vi "Unit Tester.vi"() -> ()   [LabVIEW 2012]
doc: "This VI lists all VI's in the various \"unit tests\" directories located under the directory in which this VI resides. It is then possible to run the unit tests or open the test panels. Unit tests must have a compatible connector pane for a call by reference. This user interface will be replaced by a more scripting oriented alternative in due time."
uses:
  t_Unit Tester States.ctl
panel:
  in  "open selected":bool
  in  "unit test call type":refnum<vi>
  in  "reinitialize":bool
  in  "abort":bool
  in  "run all":bool
  in  "unit tests":i32[](listbox)
  in  "stop":bool
  in  "run selected":bool
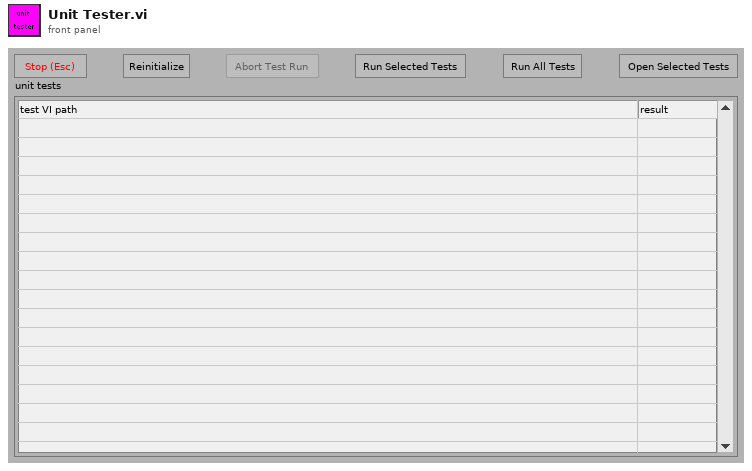
[diagram p1: front panel]
types:
  T1 = typedef "t_Unit Tester States.ctl" = enum16{"empty queue", "adjust size", "run", "open", "initialize", "cleanup", "stop"}
  T2 = enum32{"Bad", "Idle", "Run top level", "Running"}
  T3 = typedef "eventvkey.ctl" = enum16{"ASCII", "Enter", "Return", "Shift", "Ctrl", "Alt", "Cmd", "Opt", "Caps", "NumLock", "Clear", "Break", "Up", "Down", "Left", "Right", "Insert", "Delete", "Home", "End", "PageUp", "PageDown", "Escape", "Help", "Pause", "ScrollLock", "F1", "F2", "F3", "F4", "F5", "F6", "F7", "F8", "F9", "F10", "F11", "F12", "F13", "F14", "F15", "F16", "F17", "F18", "F19", "F20", "F21", "F22", "F23", "F24", "Play", "VolumeUp", "VolumeDown", "Mute", "Two Byte Char"}
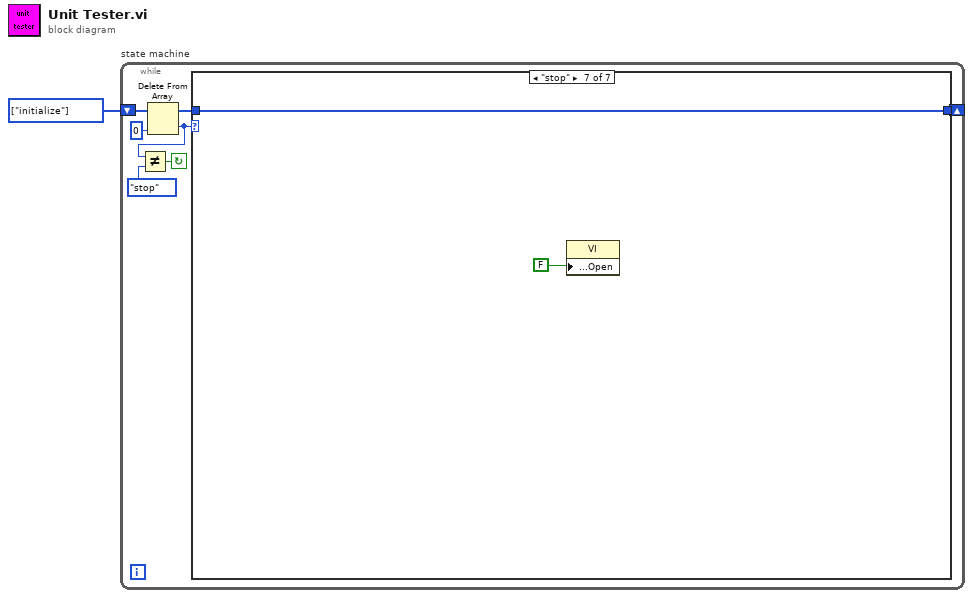
[diagram p0: block diagram]
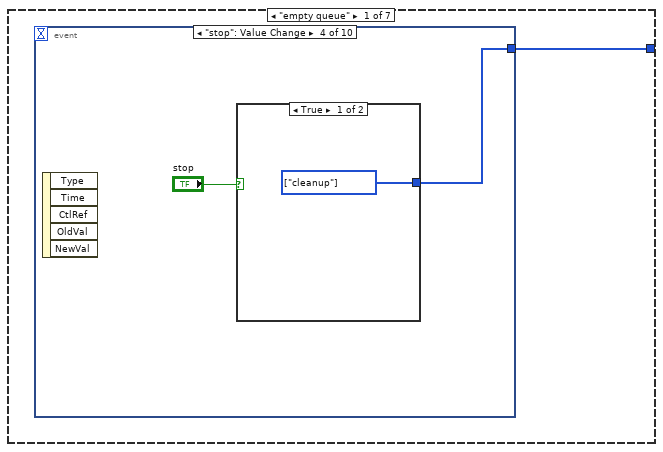
[diagram p2: hidden frame]
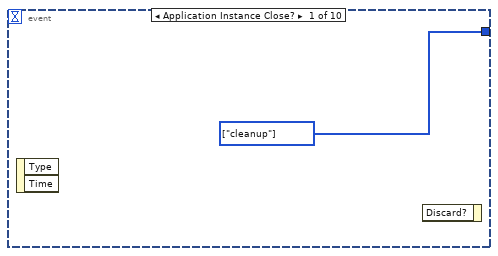
[diagram p3: hidden frame]
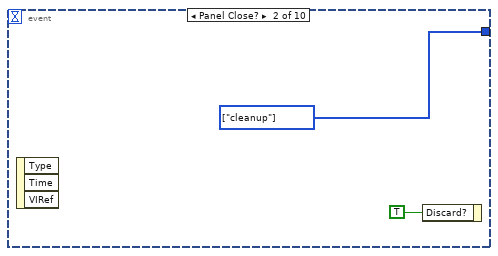
[diagram p4: hidden frame]
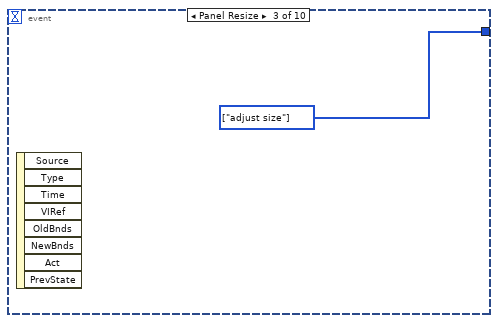
[diagram p5: hidden frame]
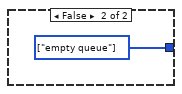
[diagram p6: hidden frame]
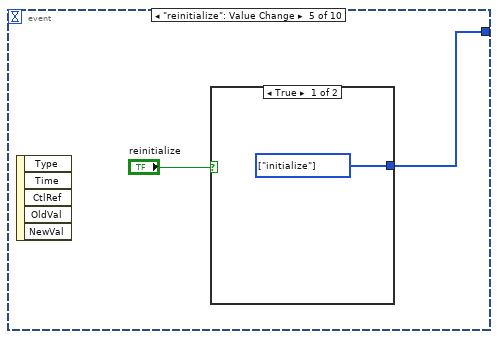
[diagram p7: hidden frame]
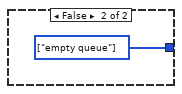
[diagram p8: hidden frame]
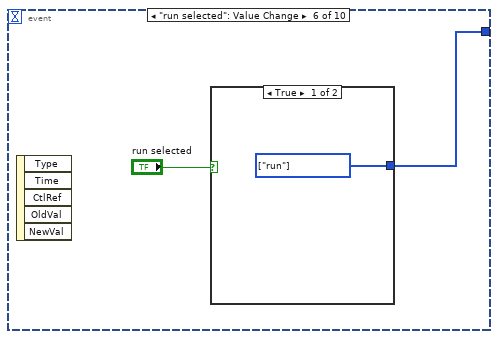
[diagram p9: hidden frame]
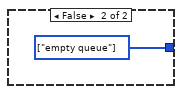
[diagram p10: hidden frame]
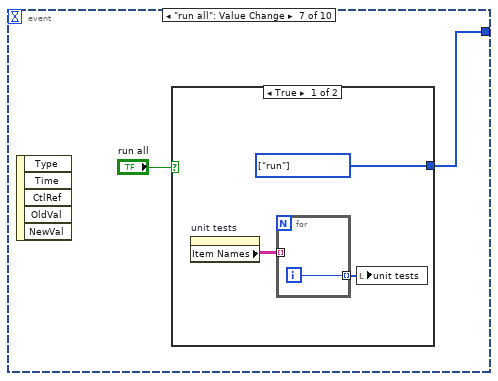
[diagram p11: hidden frame]
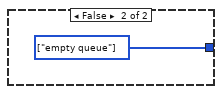
[diagram p12: hidden frame]
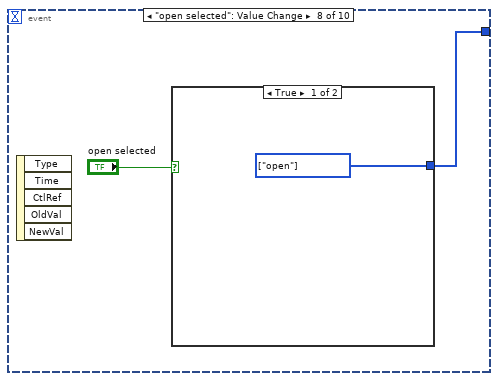
[diagram p13: hidden frame]
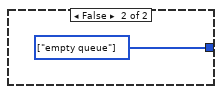
[diagram p14: hidden frame]
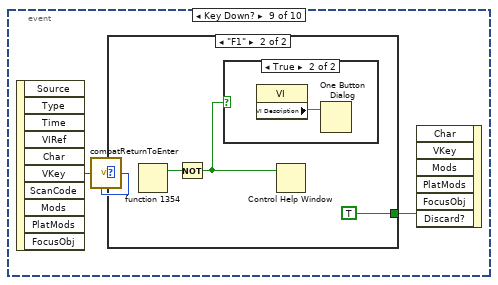
[diagram p15: hidden frame]
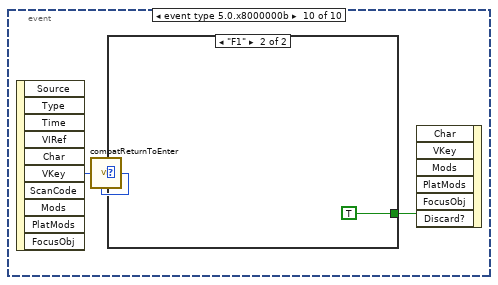
[diagram p18: hidden frame]
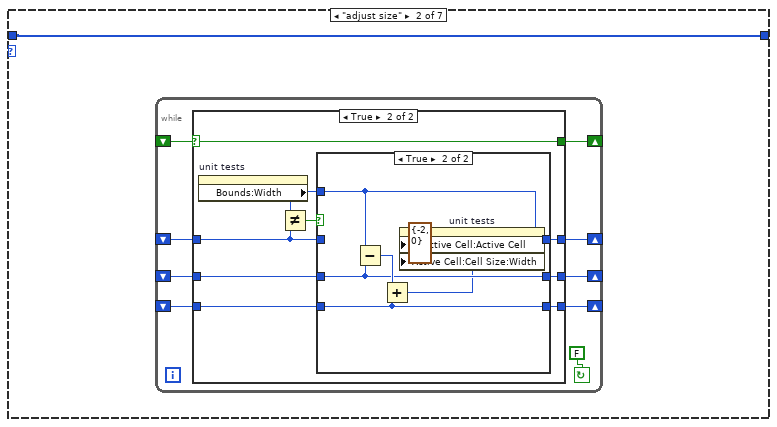
[diagram p20: hidden frame]
diagram:
  w1 = T1[] [enum."initialize"] items=["empty queue", "adjust size", "run", "open", "initialize", "cleanup", "stop"] ("Array Constant")
  n1 = while "state machine" {
    shift-left: w1 -> [w5]
    shift-right: [w8] -> _
    stop <- w7 continue-if-true
    n2 = Delete From Array(array=w5, index=0) -> (deleted portion=w3:T1, array with subset deleted=w4:T1[])  [unwired: 1 in]
    n3 = Not Equal?(x=w3, y=t_Unit_Tester_States."stop" ("states")) -> (x != y?=w7:bool)
    n4 = case "Case" shown="\"stop\"" w3 {
      tunnel: [w9 w48 w80 w142 w155 w229 w231] -> w8
      tunnel: w4 -> [_ w48 w80 w142 w171 _ w231]
      frame "empty queue" {
        n5 = event shown="[3] \"stop\": Value Change" {
          selector: _ -> [_ _ _ _ _ _ _ _ _ _]
          dyn-events: _ -> [_ _ _ _ _ _ _ _ _ _]
          timeout: _ -> [_ _ _ _ _ _ _ _ _ _]
          tunnel: [w10 w12 w13 w15 w19 w22 w27 w34 _ _] -> w9
          event Application Instance Close? {
            w10 = T1[] [enum."cleanup"] items=["empty queue", "adjust size", "run", "open", "initialize", "cleanup", "stop"] ("Array Constant")
            n6 = event-data() -> ()  [unwired: 1 in, 2 out]
            n7 = event-data() -> ()  [unwired: 2 in, 1 out]
          }
          event Panel Close? {
            w12 = T1[] [enum."cleanup"] items=["empty queue", "adjust size", "run", "open", "initialize", "cleanup", "stop"] ("Array Constant")
            n8 = event-data() -> ()  [unwired: 1 in, 3 out]
            n9 = event-data("Discard?"=TRUE) -> ()  [unwired: 1 in, 1 out]
          }
          event Panel Resize {
            w13 = T1[] [enum."adjust size"] items=["empty queue", "adjust size", "run", "open", "initialize", "cleanup", "stop"] ("Array Constant")
            n10 = event-data() -> ()  [unwired: 1 in, 8 out]
          }
          event "stop": Value Change {
            n11 = event-data() -> ()  [unwired: 1 in, 5 out]
            n12 = case shown="True" "stop" {
              tunnel: [w16 w17] -> w15
              frame True {
                w16 = T1[] [enum."cleanup"] items=["empty queue", "adjust size", "run", "open", "initialize", "cleanup", "stop"] ("Array Constant")
              }
              frame False {
                w17 = T1[] [enum."empty queue"] items=["empty queue", "adjust size", "run", "open", "initialize", "cleanup", "stop"] ("Array Constant")
              }
            }
          }
          event "reinitialize": Value Change {
            n13 = event-data() -> ()  [unwired: 1 in, 5 out]
            n14 = case shown="True" "reinitialize" {
              tunnel: [w20 w21] -> w19
              frame True {
                w20 = T1[] [enum."initialize"] items=["empty queue", "adjust size", "run", "open", "initialize", "cleanup", "stop"] ("Array Constant")
              }
              frame False {
                w21 = T1[] [enum."empty queue"] items=["empty queue", "adjust size", "run", "open", "initialize", "cleanup", "stop"] ("Array Constant")
              }
            }
          }
          event "run selected": Value Change {
            n15 = event-data() -> ()  [unwired: 1 in, 5 out]
            n16 = case shown="True" "run selected" {
              tunnel: [w24 w25] -> w22
              frame True {
                w24 = T1[] [enum."run"] items=["empty queue", "adjust size", "run", "open", "initialize", "cleanup", "stop"] ("Array Constant")
              }
              frame False {
                w25 = T1[] [enum."empty queue"] items=["empty queue", "adjust size", "run", "open", "initialize", "cleanup", "stop"] ("Array Constant")
              }
            }
          }
          event "run all": Value Change {
            n17 = event-data() -> ()  [unwired: 1 in, 5 out]
            n18 = case shown="True" "run all" {
              tunnel: [w30 w32] -> w27
              frame True {
                w30 = T1[] [enum."run"] items=["empty queue", "adjust size", "run", "open", "initialize", "cleanup", "stop"] ("Array Constant")
                n19 = property on="unit tests" class="MCListbox (strict)"() -> ("Item Names"=w29:string[][])  [unwired: 2 in, 2 out]
                n20 = for {
                  tunnel: w29 -> [_] mode=indexing
                  tunnel: [w31] -> w28 mode=indexing
                  i -> [w31]
                }
                n21 = local write "unit tests"(w28) -> ()
              }
              frame False {
                w32 = T1[] [enum."empty queue"] items=["empty queue", "adjust size", "run", "open", "initialize", "cleanup", "stop"] ("Array Constant")
              }
            }
          }
          event "open selected": Value Change {
            n22 = event-data() -> ()  [unwired: 1 in, 5 out]
            n23 = case shown="True" "open selected" {
              tunnel: [w35 w36] -> w34
              frame True {
                w35 = T1[] [enum."open"] items=["empty queue", "adjust size", "run", "open", "initialize", "cleanup", "stop"] ("Array Constant")
              }
              frame False {
                w36 = T1[] [enum."empty queue"] items=["empty queue", "adjust size", "run", "open", "initialize", "cleanup", "stop"] ("Array Constant")
              }
            }
          }
          event Key Down? {
            n24 = event-data() -> ("VKey"=w37:T3)  [unwired: 1 in, 9 out]
            n25 = call <vilib>:"compatReturnToEnter.vi"("VKey"=w37) -> ("VKey"=w39:T3)
            n26 = case shown="\"F1\"" w39 {
              tunnel: [_ TRUE] -> w38
              frame Default {
              }
              frame "F1" {
                n27 = fn#1354() -> (1:w42:bool)  [unwired: 1 out]
                n28 = Not(x=w42) -> (.not. x?=w40:bool)
                n29 = case shown="True" w40 {
                  frame False {
                  }
                  frame True {
                    n30 = property class="VI"() -> ("VI Description"=w43:string)  [unwired: 2 in, 2 out]
                    n31 = One Button Dialog(message=w43) -> ()  [unwired: 1 in, 1 out]
                  }
                }
                n32 = Control Help Window(1:w40) -> ()  [unwired: 1 in]
              }
            }
            n33 = event-data("Discard?"=w38) -> ()  [unwired: 6 in, 1 out]
          }
          event event type 5.0.x8000000b {
            n34 = event-data() -> ("VKey"=w44:T3)  [unwired: 1 in, 9 out]
            n35 = call <vilib>:"compatReturnToEnter.vi"("VKey"=w44) -> ("VKey"=w46:T3)
            n36 = case shown="\"F1\"" w46 {
              tunnel: [_ TRUE] -> w45
              frame Default {
              }
              frame "F1" {
              }
            }
            n37 = event-data("Discard?"=w45) -> ()  [unwired: 6 in, 1 out]
          }
        }
      }
      frame "adjust size" {
        n38 = while {
          shift-right: [w54] -> _
          shift-left: _ -> [w51]
          shift-right: [w55] -> _
          shift-left: _ -> [w50]
          shift-right: [w52] -> _
          shift-left: _ -> [w56]
          shift-right: [w53] -> _
          shift-left: _ -> [w49]
          stop <- FALSE continue-if-true
          n39 = case shown="True" w56 {
            selector: w56 -> [_ w70]
            tunnel: [w59 w65] -> w55
            tunnel: [w61 w63] -> w54
            tunnel: [w59 w67] -> w53
            tunnel: [TRUE w70] -> w52
            tunnel: w51 -> [_ w64]
            tunnel: w50 -> [_ w66]
            tunnel: w49 -> [_ w68]
            frame False {
              n40 = property on="unit tests" class="MulticolumnListbox (strict)"("Active Cell:Active Cell"=cluster{i32, i32} {0, 0} ("Active Cell")) -> ("Bounds:Width"=w59:u32, "Active Cell:Cell Size:Width"=w61:u32)  [unwired: 2 in, 2 out]
            }
            frame True {
              n41 = property on="unit tests" class="MulticolumnListbox (strict)"() -> ("Bounds:Width"=w62:u32)  [unwired: 2 in, 2 out]
              n42 = Not Equal?(x=w62, y=w68) -> (x != y?=w69:bool)
              n43 = case shown="True" w69 {
                tunnel: [w73 w79] -> w67
                tunnel: w68 -> [w73 _]
                tunnel: w66 -> [w72 w76]
                tunnel: [w72 w76] -> w65
                tunnel: w64 -> [w71 w74]
                tunnel: [w71 w74] -> w63
                tunnel: w62 -> [_ w79]
                frame False {
                }
                frame True {
                  n44 = Subtract(x=w79, y=w76) -> (x-y=w78:u32)
                  n45 = Add(x=w78, y=w74) -> (x+y=w75:u32)
                  n46 = property on="unit tests" class="MulticolumnListbox (strict)"("Active Cell:Active Cell"=cluster{i32, i32} {-2, 0} ("Active Cell"), "Active Cell:Cell Size:Width"=w75) -> ()  [unwired: 2 in, 2 out]
                }
              }
            }
          }
        }
      }
      frame "run" {
        n47 = stacked-sequence {
          frame #0 {
            w81 = u8 1 items=["enabled", "disabled", "grayed"] ("disabled state")
            w82 = u8 2 items=["enabled", "disabled", "grayed"] ("disabled state")
            w83 = u8 0 items=["enabled", "disabled", "grayed"] ("disabled state")
            n48 = property on="unit tests" class="MCListbox (strict)"("Disabled"=w81) -> ()  [unwired: 2 in, 2 out]
            n49 = property on="stop" class="Bool"("Disabled"=w82) -> ()  [unwired: 2 in, 2 out]
            n50 = property on="reinitialize" class="Bool"("Disabled"=w82) -> ()  [unwired: 2 in, 2 out]
            n51 = property on="run selected" class="Bool"("Disabled"=w82) -> ()  [unwired: 2 in, 2 out]
            n52 = property on="run all" class="Bool"("Disabled"=w82) -> ()  [unwired: 2 in, 2 out]
            n53 = property on="open selected" class="Bool"("Disabled"=w82) -> ()  [unwired: 2 in, 2 out]
            n54 = property on="abort" class="Bool"("Disabled"=w83) -> ()  [unwired: 2 in, 2 out]
          }
          frame #1 {
            n55 = property on="unit tests" class="MCListbox (strict)"() -> ("Item Names"=w86:string[][])  [unwired: 2 in, 2 out]
            n56 = Array Size(array="unit tests") -> (size(s)=w85:i32)
            n57 = case shown="Default" w85 {
              tunnel: "unit tests" -> [_ w88]
              tunnel: w86 -> [_ w87]
              frame 0 {
              }
              frame Default {
                n58 = while {
                  shift-right: [w98] -> _
                  shift-left: w88 -> [w109]
                  shift-right: [w101] -> _
                  shift-left: w87 -> [w100]
                  stop <- w99 stop-if-true
                  n59 = Delete From Array(array=w109, index=0) -> (deleted portion=w92:i32, array with subset deleted=w98:i32[])  [unwired: 1 in]
                  n60 = Index Array(array=w100, index (row)=w92, index (col)=0 ("disabled index (col)")) -> (element=w107:string)
                  n61 = String To Path(string=w107) -> (path=w105:path)
                  n62 = Open VI Reference(type specifier VI Refnum (for type only)="unit test call type", vi path=w105) -> (vi reference=w102:refnum<vi>, error out=w104:errorcluster)  [unwired: 4 in]
                  n63 = case shown="No Error" w104 {
                    tunnel: w102 -> [w124 _]
                    tunnel: [w117 "Load error"] -> w96
                    frame No Error {
                      n64 = property class="cached class 0"(reference=w124) -> (reference out=w120:refnum<vi>, error out=w118:errorcluster, "Execution:State"=w122:T2)  [unwired: 1 in]
                      n65 = Equal?(x=w122, y=T2."Bad" ("Execution:State")) -> (x = y?=w121:bool)
                      n66 = case shown="False" w121 {
                        tunnel: w120 -> [w134 w136]
                        tunnel: [w132 w136] -> w119
                        tunnel: [w126 "Broken"] -> w117
                        tunnel: w118 -> [w133 _]
                        frame False {
                          n67 = call-by-ref "?"(reference=w134, error in=w133) -> (reference out=w132:refnum<vi>, error out=w128:errorcluster, "pass?"=w125:bool)  [unwired: 1 in]
                          n68 = Select(t="Pass", s=w125, f="Fail") -> (s? t:f=w131:string)
                          n69 = Select(t="Run Error", s=w128, f=w131) -> (s? t:f=w126:string)
                        }
                        frame True {
                        }
                      }
                      n70 = Close Reference(reference=w119) -> ()  [unwired: 1 in, 1 out]
                    }
                    frame Error {
                    }
                  }
                  n71 = Not Equal?(x=w96, y="Pass") -> (x != y?=w91:bool)
                  n72 = Bundle(w92, "element"=1) -> (w90:cluster{i32, "element":i32})  [unwired: 1 in]
                  n73 = Select(t=u32 16727100, s=w91, f=u32 15790320) -> (s? t:f=w89:u32)
                  n74 = property on="unit tests" class="MCListbox (strict)"("Active Cell:Active Cell"=w90, "Active Cell:Cell Background Color"=w89) -> ()  [unwired: 2 in, 2 out]
                  n75 = Replace Array Subset(array=w100, new element=w96, index (row)=w92, index (col)=1 ("disabled index (col)")) -> (w101:string[][])
                  n76 = stacked-sequence {
                    tunnel: [w113] -> w99
                    tunnel: w98 -> [w112]
                    tunnel: w101 -> [w111]
                    frame #0 {
                      n77 = Array Size(array=w112) -> (size(s)=w116:i32)
                      n78 = local write "unit tests"(w112) -> ()
                      n79 = Equal To 0?(x=w116) -> (x = 0?=w115:bool)
                      n80 = Or(x=w115, y="abort") -> (x .or. y?=w113:bool)
                      n81 = property on="unit tests" class="MCListbox (strict)"("Item Names"=w111) -> ()  [unwired: 2 in, 2 out]
                    }
                  }
                }
              }
            }
          }
          frame #2 {
            w139 = u8 2 items=["enabled", "disabled", "grayed"] ("disabled state")
            w138 = u8 0 items=["enabled", "disabled", "grayed"] ("disabled state")
            n82 = property on="abort" class="Bool"("Disabled"=w139) -> ()  [unwired: 2 in, 2 out]
            n83 = property on="unit tests" class="MCListbox (strict)"("Disabled"=w138) -> ()  [unwired: 2 in, 2 out]
            n84 = property on="stop" class="Bool"("Disabled"=w138) -> ()  [unwired: 2 in, 2 out]
            n85 = property on="reinitialize" class="Bool"("Disabled"=w138) -> ()  [unwired: 2 in, 2 out]
            n86 = property on="run selected" class="Bool"("Disabled"=w138) -> ()  [unwired: 2 in, 2 out]
            n87 = property on="run all" class="Bool"("Disabled"=w138) -> ()  [unwired: 2 in, 2 out]
            n88 = property on="open selected" class="Bool"("Disabled"=w138) -> ()  [unwired: 2 in, 2 out]
          }
        }
      }
      frame "open" {
        n89 = property on="unit tests" class="MCListbox (strict)"() -> ("Item Names"=w141:string[][])  [unwired: 2 in, 2 out]
        n90 = local read "unit tests"() -> (w140:i32[])
        n91 = for {
          tunnel: w141 -> [w147]
          tunnel: w140 -> [w143] mode=indexing
          n92 = Index Array(array=w147, index (row)=w143, index (col)=0 ("disabled index (col)")) -> (element=w150:string)
          n93 = String To Path(string=w150) -> (path=w149:path)
          n94 = Open VI Reference(vi path=w149) -> (vi reference=w148:refnum<vi>, error out=w146:errorcluster)  [unwired: 5 in]
          n95 = property class="VI"(reference=w148, error in=w146, "Front Panel Window:Open"=TRUE) -> (reference out=w144:refnum<vi>)  [unwired: 1 out]
          n96 = Close Reference(reference=w144) -> ()  [unwired: 1 in, 1 out]
        }
      }
      frame "initialize" {
        w156 = -2 ("element")
        w166 = 0 ("dimension size")
        # "avoid LV7 bug"
        n97 = Current VI's Path() -> (path=w170:path)
        n98 = Strip Path(path=w170) -> (stripped path=w160:path)  [unwired: 1 out]
        n99 = Bundle("element"=w156, "element"=w156) -> (w157:cluster{"element":i32, "element":i32})  [unwired: 1 in]
        n100 = Build Array(w160) -> (w162:path[])
        n101 = property on="unit tests" class="MCListbox (strict)"("Active Cell:Active Cell"=w157, "Active Cell:Cell Background Color"=u32 15790320) -> ()  [unwired: 2 in, 2 out]
        n102 = while "recursively list directories" {
          shift-left: errorcluster {"status"=FALSE, "code"=0, "source"=""} ("error IO") -> [w184]
          shift-right: [w175] -> w161
          shift-left: w162 -> [w180]
          shift-right: [w179] -> w152
          i -> [w178]
          stop <- w172 stop-if-true
          n103 = Index Array(array=w180, index=w178) -> (element=w182:path)
          n104 = List Folder(path=w182, error in=w184) -> (folder names=w183:string[], error out=w181:errorcluster)  [unwired: 2 in, 2 out]
          n105 = case shown="No Error" w181 {
            selector: w181 -> [w185 w194]
            tunnel: w183 -> [w190 _]
            tunnel: w182 -> [w189 _]
            tunnel: w180 -> [w188 w195]
            tunnel: [w186 w195] -> w179
            tunnel: [w185 w194] -> w175
            frame No Error {
              n106 = for {
                tunnel: w190 -> [w192] mode=indexing
                tunnel: w189 -> [w193]
                tunnel: [w191] -> w187 mode=indexing
                n107 = Build Path(base path=w193, name or relative path=w192) -> (appended path=w191:path)
              }
              n108 = Build Array (concatenate)(w188, w187) -> (w186:path[])
            }
            frame Error {
            }
          }
          n109 = Array Size(array=w179) -> (size(s)=w177:i32)
          n110 = Increment(x=w178) -> (x+1=w176:i32)
          n111 = Less Or Equal?(x=w177, y=w176) -> (x <= y?=w174:bool)
          n112 = Unbundle By Name(w175) -> ("status"=w173:bool)
          n113 = Or(x=w173, y=w174) -> (x .or. y?=w172:bool)
        }
        n114 = Sort 1D Array(array=w152) -> (sorted array=w153:path[])
        n115 = Sort 1D Array(array=w153) -> (sorted array=w163:path[])
        n116 = Initialize Array("", w166, w166) -> (w167:string[][])
        n117 = for "collect all unit tests (files in directories named \"unit tests\")" {
          tunnel: w163 -> [w200] mode=indexing
          shift-right: [w198] -> w169
          shift-left: w161 -> [w199]
          shift-right: [w196] -> w165
          shift-left: w167 -> [w197]
          n118 = Strip Path(path=w200) -> (name=w204:string)  [unwired: 1 out]
          n119 = To Lower Case(string=w204) -> (all lower case string=w202:string)
          n120 = Equal?(x="unit tests", y=w202) -> (x = y?=w201:bool)
          n121 = case shown="True" w201 {
            tunnel: w200 -> [_ w216]
            tunnel: w199 -> [w206 w215]
            tunnel: [w206 w211] -> w198
            tunnel: w197 -> [w205 w212]
            tunnel: [w205 w210] -> w196
            frame False {
            }
            frame True {
              # "avoid LV7 bug"
              n122 = List Folder(path=w216, error in=w215) -> (path out=w213:path, filenames=w209:string[], error out=w214:errorcluster)  [unwired: 2 in, 1 out]
              n123 = Sort 1D Array(array=w209) -> (sorted array=w208:string[])
              n124 = Sort 1D Array(array=w208) -> (sorted array=w207:string[])
              n125 = for {
                shift-right: [w220] -> w211
                shift-left: w214 -> [w220]
                tunnel: w213 -> [w224]
                tunnel: w207 -> [w225] mode=indexing
                shift-right: [w221] -> w210
                shift-left: w212 -> [w222]
                n126 = Build Path(base path=w224, name or relative path=w225) -> (appended path=w223:path)
                n127 = Path To String(path=w223) -> (string=w219:string)
                n128 = Build Array(w219, "") -> (w217:string[])
                n129 = Build Array (concatenate)(w222, w217) -> (w221:string[][])
              }
            }
          }
        }
        n130 = local write "unit tests"(i32[] [] ("unit tests")) -> ()
        n131 = property on="unit tests" class="MCListbox (strict)"("Item Names"=w165) -> ()  [unwired: 2 in, 2 out]
        n132 = call "Library Log Error to Window.vi"("error in (no error)"=w169) -> ()  [unwired: 13 in, 2 out]
        n133 = Build Array (concatenate)(w171, t_Unit_Tester_States."adjust size" ("states")) -> (w155:T1[])
      }
      frame "cleanup" {
        w227 = u8 2 items=["enabled", "disabled", "grayed"] ("disabled state")
        w228 = u8 0 items=["enabled", "disabled", "grayed"] ("disabled state")
        w229 = T1[] [enum."stop"] items=["empty queue", "adjust size", "run", "open", "initialize", "cleanup", "stop"] ("Array Constant")
        n134 = property on="unit tests" class="MCListbox (strict)"("Item Names"=string[][] []) -> ()  [unwired: 2 in, 2 out]
        n135 = property on="abort" class="Bool"("Disabled"=w227) -> ()  [unwired: 2 in, 2 out]
        n136 = property on="unit tests" class="MCListbox (strict)"("Disabled"=w228) -> ()  [unwired: 2 in, 2 out]
        n137 = property on="stop" class="Bool"("Disabled"=w228) -> ()  [unwired: 2 in, 2 out]
        n138 = property on="reinitialize" class="Bool"("Disabled"=w228) -> ()  [unwired: 2 in, 2 out]
        n139 = property on="run selected" class="Bool"("Disabled"=w228) -> ()  [unwired: 2 in, 2 out]
        n140 = property on="run all" class="Bool"("Disabled"=w228) -> ()  [unwired: 2 in, 2 out]
        n141 = property on="open selected" class="Bool"("Disabled"=w228) -> ()  [unwired: 2 in, 2 out]
      }
      frame "stop" {
        n142 = property class="VI"("Front Panel Window:Open"=FALSE) -> ()  [unwired: 2 in, 2 out]
      }
    }
  }
